vi "Teleop.vi"(10 "Match Info":T1={"Autonomous Elapsed Seconds"=0.0, "TeleOp Elapsed Seconds"=0.0, "Disabled Elapsed Seconds"=0.0, "Visited Autonomous"=FALSE, "Visited TeleOp"=FALSE, "Visited Disabled"=FALSE, "Autonomous Settings"={"Autonomous Style"=enum."Independent", "VI Refnum"=refnum}}, 11 "Call Context":T2) -> ()   [LabVIEW 2015]
doc: "This VI is called for each TeleOp packet received from the DS where the robot is not disabled. It is often used to read from the joysticks and update I/O or to update setpoints for timed control loops. It should complete and return within 20 milliseconds or it may miss DS packets."
uses:
  <vilib>/Rock Robotics/WPI/DriverStation/WPI_DriverStationDerivedRobotMode.ctl
  <vilib>/Rock Robotics/WPI/DriverStation/WPI_DriverStationMatch Info.ctl
  <vilib>/Rock Robotics/WPI/Utilities/WPI_GetSetVariantRefNum.vi
  <vilib>/Rock Robotics/Network Tables/NT Write Boolean Array.vi
  <vilib>/Rock Robotics/Network Tables/NT Write Numeric Array.vi
  <vilib>/Rock Robotics/Network Tables/NT Write Boolean.vi
  <vilib>/Rock Robotics/Network Tables/NT Write Number.vi
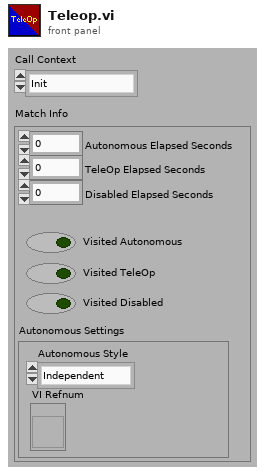
[diagram p1: front panel]
types:
  T1 = typedef "WPI_DriverStationMatch Info.ctl" = cluster{"Autonomous Elapsed Seconds":dbl, "TeleOp Elapsed Seconds":dbl, "Disabled Elapsed Seconds":dbl, "Visited Autonomous":bool, "Visited TeleOp":bool, "Visited Disabled":bool, "Autonomous Settings":cluster{"Autonomous Style":enum16{"Iterative", "Independent"}, "VI Refnum":refnum<vi>}}
  T2 = typedef "WPI_DriverStationDerivedRobotMode.ctl" = enum16{"Init", "Execute", "Stop"}
  T3 = typedef "WPI_JoystickDevRef.ctl" = cluster{"Device":T4}
  T4 = typedef "WPI_JoystickDeviceEnum.ctl" = enum16{"USB 0", "USB 1", "USB 2", "USB 3", "USB 4", "USB 5"}
  T5 = typedef "WPI_EncoderDevRef.ctl" = cluster{"DevStatus":errorcluster, "EncoderIndex":T6, "CounterIndex":T7, "DistancePerCount":dbl, "Decoding Type":T8}
  T6 = typedef "FPGA_EncoderIdx.ctl" = enum8{"Enc 0", "Enc 1", "Enc 2", "Enc 3", "Enc 4", "Enc 5", "Enc 6", "Enc 7", "Invalid"}
  T7 = typedef "FPGA_CounterCtrSystemIndex.ctl" = enum8{"Ctr 0", "Ctr 1", "Ctr 2", "Ctr 3", "Ctr 4", "Ctr 5", "Ctr 6", "Ctr 7", "Invalid"}
  T8 = typedef "WPI_EncoderType.ctl" = enum16{"1x", "2x", "4x"}
  T9 = typedef "WPI_RobotDriveDevRef.ctl" = cluster{"DevStatus":errorcluster, "Motors[]":T10[], "Square Inputs":bool, "Max Output":dbl}
  T10 = typedef "WPI_MotorControlDeviceRef.ctl" = cluster{"DeviceStatus":errorcluster, "Type":T11, "PWM":cluster{"PWM Channel":T12, "DeadBand":T13}, "CAN":cluster{"Device Number":u8, "Control Mode":T14, "Semaphore":T15, "Max Vout":dbl, "TalonSRX Control Mode":T16}, "Invert":bool}
  T11 = typedef "WPI_MotorControlType.ctl" = enum16{"PWM", "CAN", "CANTalonSRX"}
  T12 = typedef "FPGA_DIOPWMChannel.ctl" = enum8{"PWM 0", "PWM 1", "PWM 2", "PWM 3", "PWM 4", "PWM 5", "PWM 6", "PWM 7", "PWM 8", "PWM 9", "PWM MXP 0", "PWM MXP 1", "PWM MXP 2", "PWM MXP 3", "PWM MXP 4", "PWM MXP 5", "PWM MXP 6", "PWM MXP 7", "PWM MXP 8", "PWM MXP 9", "Invalid"}
  T13 = typedef "WPI_PWMDeadband.ctl" = cluster{"Name":string, "maxPositivePwm":i32, "minPositivePwm":i32, "centerPwm":i32, "maxNegativePwm":i32, "minNegativePwm":i32, "angularRange":u16}
  T14 = typedef "WPI_CANJaguar_ControlMode.ctl" = enum8{"Percent VBus", "Current", "Speed", "Position", "Voltage"}
  T15 = typedef "Semaphore RefNum" = refnum<k1>
  T16 = typedef "WPI_CANTalonSRX_APIControlMode.ctl" = enum8{"Percent VBus", "Speed", "Position", "Slave", "Unchanged / Invalid", "Voltage Compensation", "Current", "Motion Profile"}
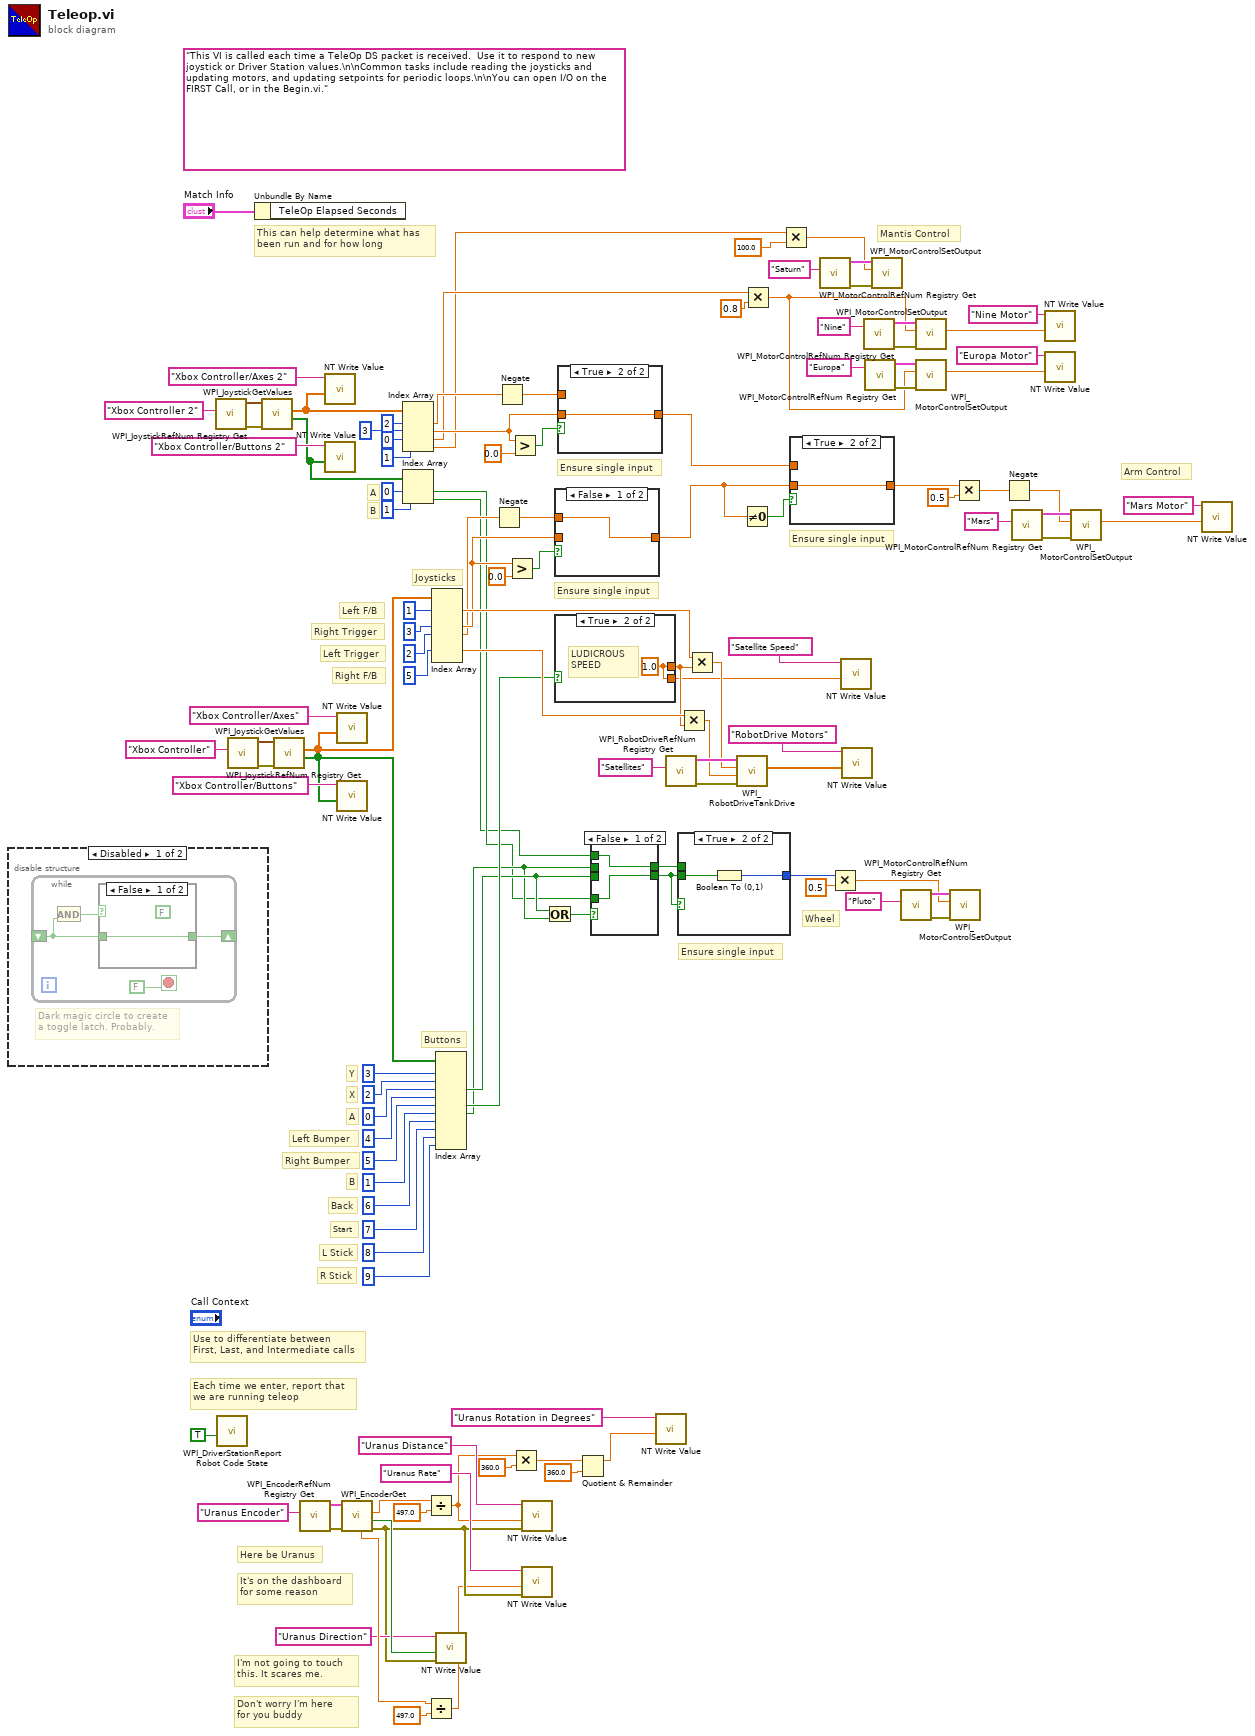
[diagram p0: block diagram]
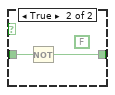
[diagram p5: hidden frame]
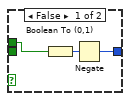
[diagram p7: hidden frame]
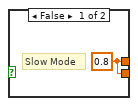
[diagram p9: hidden frame]
diagram:
  (unwired) "This VI is called each time a TeleOp DS packet is received.  Use it to respond to new joystick or Driver Station values.\n\nCommon tasks include reading the joysticks and updating motors, and updating setpoints for periodic loops.\n\nYou can open I/O on the FIRST Call, or in the Begin.vi."
  # "Mantis Control"
  # "B"
  # "A"
  # "Ensure single input"
  # "Ensure single input"
  # "R Stick"
  # "L Stick"
  # "Start"
  # "Back"
  # "X"
  # "B"
  # "A"
  # "Don't worry I'm here    \nfor you buddy"
  # "I'm not going to touch\nthis. It scares me."
  # "It's on the dashboard\nfor some reason"
  # "Here be Uranus"
  # "Ensure single input"
  # "Ensure single input"
  # "Wheel"
  # "Arm Control"
  # "Buttons"
  # "Y"
  # "Right Bumper"
  # "Left Bumper"
  # "Joysticks"
  # "Right F/B"
  # "Left Trigger"
  # "Right Trigger"
  # "Left F/B"
  # "Each time we enter, report that\nwe are running teleop"
  # "Use to differentiate between\nFirst, Last, and Intermediate calls"
  # "This can help determine what has\nbeen run and for how long"
  n1 = disable-structure shown="Disabled" {
    frame Disabled {
      # "Dark magic circle to create\na toggle latch. Probably."
      n2 = while {
        shift-right: [w125] -> _
        shift-left: _ -> [w124]
        stop <- FALSE stop-if-true
        n3 = And(y=w124) -> (x .and. y?=w123:bool)  [unwired: 1 in]
        n4 = case shown="False" w123 {
          tunnel: w124 -> [w127 w129]
          tunnel: [w127 w128] -> w125
          frame False {
            (unwired) FALSE
          }
          frame True {
            (unwired) FALSE
            n5 = Not(x=w129) -> (.not. x?=w128:bool)
          }
        }
      }
    }
    frame Enabled {
    }
  }
  n6 = call <vilib>:"WPI_JoystickRefNum Registry Get.vi"("refnum name"="Xbox Controller 2") -> ("error out"=w41:errorcluster, "JoystickDevRef"=w44:T3)  [unwired: 1 in, 8 out]
  n7 = call <vilib>:"WPI_DriverStationReport Robot Code State.vi"("TeleOp"=TRUE ("Autonomous")) -> ()  [unwired: 10 in, 1 out]
  n8 = call <vilib>:"WPI_JoystickRefNum Registry Get.vi"("refnum name"="Xbox Controller") -> ("error out"=w94:errorcluster, "JoystickDevRef"=w118:T3)  [unwired: 1 in, 8 out]
  n9 = Unbundle By Name("Match Info") -> ()  [unwired: 1 out]
  n10 = call <vilib>:"WPI_JoystickGetValues.vi"("error in (no error)"=w41, "JoystickDevRef"=w44) -> ("Buttons"=w32:bool[], "Axes"=w39:dbl[])  [unwired: 5 in, 3 out]
  n11 = call <vilib>:"WPI_JoystickGetValues.vi"("error in (no error)"=w94, "JoystickDevRef"=w118) -> ("Buttons"=w56:bool[], "Axes"=w57:dbl[])  [unwired: 5 in, 3 out]
  n12 = call <vilib>:"WPI_EncoderRefNum Registry Get.vi"("refnum name"="Uranus Encoder") -> ("error out"=w109:errorcluster, "EncoderDevRef"=w108:T5)  [unwired: 9 in]
  n13 = call-poly <vilib>:"NT Write Value.vi"("Numeric Array"=w39, "Name"="Xbox Controller/Axes 2") -> ()  [unwired: 9 in, 1 out]
  n14 = call-poly <vilib>:"NT Write Value.vi"("Boolean Array"=w32, "Name"="Xbox Controller/Buttons 2") -> ()  [unwired: 9 in, 1 out]
  n15 = call-poly <vilib>:"NT Write Value.vi"("Numeric Array"=w57, "Name"="Xbox Controller/Axes") -> ()  [unwired: 9 in, 1 out]
  n16 = call-poly <vilib>:"NT Write Value.vi"("Boolean Array"=w56, "Name"="Xbox Controller/Buttons") -> ()  [unwired: 9 in, 1 out]
  n17 = call <vilib>:"WPI_EncoderGet.vi"("error in (no error)"=w109, "EncoderDevRef"=w108) -> ("error out"=w101:errorcluster, "Direction"=w106:bool, "Distance"=w107:dbl, "Rate"=w105:dbl)  [unwired: 4 in, 2 out]
  n18 = Index Array(array=w39, index #1=2 ("index"), index #2=3 ("index"), index #3=0 ("index"), index #4=1 ("index")) -> (element #1=w40:dbl, element #2=w38:dbl, element #3=w9:dbl, element #4=w2:dbl)
  n19 = Index Array(array=w32, index #1=0 ("index"), index #2=1 ("index")) -> (element #1=w24:bool, element #2=w23:bool)
  n20 = Divide(x=w107, y=497.0) -> (x/y=w97:dbl)
  n21 = Divide(x=w105, y=497.0) -> (x/y=w100:dbl)
  n22 = Index Array(array=w57, index #1=1 ("index"), index #3=3 ("index"), index #4=2 ("index"), index #6=5 ("index")) -> (element #1=w78:dbl, element #3=w63:dbl, element #4=w61:dbl, element #6=w80:dbl)  [unwired: 3 in, 3 out]
  n23 = Index Array(array=w56, index #1=3 ("index"), index #2=2 ("index"), index #3=0 ("index"), index #4=4 ("index"), index #5=5 ("index"), index #6=1 ("index"), index #7=6 ("index"), index #8=7 ("index"), index #9=8 ("index"), index #10=9 ("index")) -> (element #3=w27:bool, element #5=w55:bool, element #6=w26:bool)  [unwired: 7 out]
  n24 = call-poly <vilib>:"NT Write Value.vi"("error in"=w101, "Boolean"=w106, "Name"="Uranus Direction") -> ()  [unwired: 8 in, 1 out]
  n25 = Negate(x=w61) -> (-x=w54:dbl)
  n26 = Negate(x=w40) -> (-x=w46:dbl)
  n27 = Greater?(x=w63, y=0.0) -> (0:w62:bool)
  n28 = Greater?(x=w38, y=0.0) -> (0:w48:bool)
  n29 = Multiply(x=w97, y=360.0) -> (x*y=w92:dbl)
  n30 = call-poly <vilib>:"NT Write Value.vi"("error in"=w101, "Numeric"=w97, "Name"="Uranus Distance") -> ()  [unwired: 8 in, 1 out]
  n31 = call-poly <vilib>:"NT Write Value.vi"("error in"=w101, "Numeric"=w100, "Name"="Uranus Rate") -> ()  [unwired: 8 in, 1 out]
  n32 = Or(x=w27, y=w26) -> (x .or. y?=w25:bool)
  n33 = case shown="False" w62 {
    tunnel: [w130 w131] -> w33
    tunnel: w63 -> [_ w131]
    tunnel: w54 -> [w130 _]
    frame False {
    }
    frame True {
    }
  }
  n34 = case shown="True" w55 {
    tunnel: [w132 w133] -> w77
    tunnel: [w132 w133] -> w76
    frame False {
      w132 = 0.8 ("y")
      # "Slow Mode"
    }
    frame True {
      w133 = 1.0 ("y")
      # "LUDICROUS \nSPEED"
    }
  }
  n35 = case shown="True" w48 {
    tunnel: [w134 w135] -> w35
    tunnel: w38 -> [_ w135]
    tunnel: w46 -> [w134 _]
    frame False {
    }
    frame True {
    }
  }
  n36 = Quotient & Remainder(x=w92, y=360.0) -> (x-y*floor(x/y)=w90:dbl)  [unwired: 1 out]
  n37 = case shown="False" w25 {
    tunnel: [w136 w139] -> w29
    tunnel: [w137 w138] -> w28
    tunnel: w27 -> [_ w138]
    tunnel: w26 -> [_ w139]
    tunnel: w24 -> [w137 _]
    tunnel: w23 -> [w136 _]
    frame False {
    }
    frame True {
    }
  }
  n38 = call-poly <vilib>:"NT Write Value.vi"("Numeric"=w90, "Name"="Uranus Rotation in Degrees") -> ()  [unwired: 9 in, 1 out]
  n39 = call <vilib>:"WPI_RobotDriveRefNum Registry Get.vi"("refnum name"="Satellites") -> ("error out"=w93:errorcluster, "RobotDriveDevRef"=w120:T9)  [unwired: 1 in, 8 out]
  n40 = case shown="True" w28 {
    tunnel: [w141 w144] -> w60
    tunnel: w28 -> [_ w143]
    tunnel: w29 -> [w140 _]
    frame False {
      n41 = Boolean To (0,1)(Boolean=w140) -> (0, 1=w142:i16)
      n42 = Negate(x=w142) -> (-x=w141:i16)
    }
    frame True {
      n43 = Boolean To (0,1)(Boolean=w143) -> (0, 1=w144:i16)
    }
  }
  n44 = Multiply(x=w80, y=w77) -> (x*y=w81:dbl)
  n45 = Multiply(x=w78, y=w77) -> (x*y=w79:dbl)
  n46 = call <vilib>:"WPI_RobotDriveTankDrive.vi"("error in (no error)"=w93, "Right axis value"=w81, "Left axis value"=w79, "RobotDriveDevRef"=w120) -> ("Motor Values"=w114:dbl[])  [unwired: 5 in, 2 out]
  n47 = Not Equal To 0?(x=w33) -> (x != 0?=w22:bool)
  n48 = Multiply(x=w9, y=0.8) -> (x*y=w10:dbl)
  n49 = Multiply(x=w2, y=100.0) -> (x*y=w3:dbl)
  n50 = case shown="True" w22 {
    tunnel: [w145 w146] -> w34
    tunnel: w33 -> [_ w146]
    tunnel: w35 -> [w145 _]
    frame False {
    }
    frame True {
    }
  }
  n51 = call <vilib>:"WPI_MotorControlRefNum Registry Get.vi"("refnum name"="Saturn") -> ("error out"=w6:errorcluster, "MotorControlDevRef"=w5:T10)  [unwired: 9 in]
  n52 = Multiply(x=w60, y=0.5) -> (x*y=w65:dbl)
  n53 = call-poly <vilib>:"NT Write Value.vi"("Numeric"=w76, "Name"="Satellite Speed") -> ()  [unwired: 9 in, 1 out]
  n54 = call-poly <vilib>:"NT Write Value.vi"("Numeric Array"=w114, "Name"="RobotDrive Motors") -> ()  [unwired: 9 in, 1 out]
  n55 = call <vilib>:"WPI_MotorControlRefNum Registry Get.vi"("refnum name"="Nine") -> ("error out"=w20:errorcluster, "MotorControlDevRef"=w19:T10)  [unwired: 9 in]
  n56 = call <vilib>:"WPI_MotorControlRefNum Registry Get.vi"("refnum name"="Europa") -> ("error out"=w15:errorcluster, "MotorControlDevRef"=w14:T10)  [unwired: 9 in]
  n57 = call <vilib>:"WPI_MotorControlSetOutput.vi"("error in (no error)"=w6, "Output"=w3, "MotorControlDevRef"=w5) -> ()  [unwired: 6 in, 3 out]
  n58 = call <vilib>:"WPI_MotorControlRefNum Registry Get.vi"("refnum name"="Pluto") -> ("error out"=w73:errorcluster, "MotorControlDevRef"=w72:T10)  [unwired: 9 in]
  n59 = call <vilib>:"WPI_MotorControlSetOutput.vi"("error in (no error)"=w20, "Output"=w10, "MotorControlDevRef"=w19) -> ("Motor Output"=w21:dbl)  [unwired: 6 in, 2 out]
  n60 = call <vilib>:"WPI_MotorControlSetOutput.vi"("error in (no error)"=w15, "Output"=w10, "MotorControlDevRef"=w14) -> ("Motor Output"=w16:dbl)  [unwired: 6 in, 2 out]
  n61 = call <vilib>:"WPI_MotorControlSetOutput.vi"("error in (no error)"=w73, "Output"=w65, "MotorControlDevRef"=w72) -> ()  [unwired: 6 in, 3 out]
  n62 = Multiply(x=w34, y=0.5) -> (x*y=w67:dbl)
  n63 = Negate(x=w67) -> (-x=w74:dbl)
  n64 = call <vilib>:"WPI_MotorControlRefNum Registry Get.vi"("refnum name"="Mars") -> ("error out"=w87:errorcluster, "MotorControlDevRef"=w86:T10)  [unwired: 9 in]
  n65 = call-poly <vilib>:"NT Write Value.vi"("Numeric"=w21, "Name"="Nine Motor") -> ()  [unwired: 9 in, 1 out]
  n66 = call-poly <vilib>:"NT Write Value.vi"("Numeric"=w16, "Name"="Europa Motor") -> ()  [unwired: 9 in, 1 out]
  n67 = call <vilib>:"WPI_MotorControlSetOutput.vi"("error in (no error)"=w87, "Output"=w74, "MotorControlDevRef"=w86) -> ("Motor Output"=w88:dbl)  [unwired: 6 in, 2 out]
  n68 = call-poly <vilib>:"NT Write Value.vi"("Numeric"=w88, "Name"="Mars Motor") -> ()  [unwired: 9 in, 1 out]
